vi "VI Algebraic Konfig.vi"() -> ()   [LabVIEW 2020, in "FT-IR.lvlib" / "Algebraic Modul.lvlib"]
uses:
  Algebraic Modul.lvlib
  Visualisierungs Elemente/Button.ctl
  FGV Algebraic Aktionen.ctl
  Messdaten/Aktionen FGV Messdaten.ctl
  FGV FT-IR Gasliste Aktionen.ctl
  FT-IR.lvlib
  Messdaten/Messdaten.lvlib
  Log Konfig/LogKonfig.lvlib
  Allgemein/allgemeine Sub-VIs.lvlib
panel:
  out "OK?":bool[](array[boolean]) caption="Gültig?"
  in  "Abbrechen":T1
  out "Aktuelle Gasliste":string[](array[string])
  in  "Formel":string[](array[string])
  in  "Namen":string[](array[string])
  in  "Speichern":T1
  # "Algebraic Konfiguration"
  # "Gasliste"
  # "Name"
  # "Formel"
  # "Gültig?"
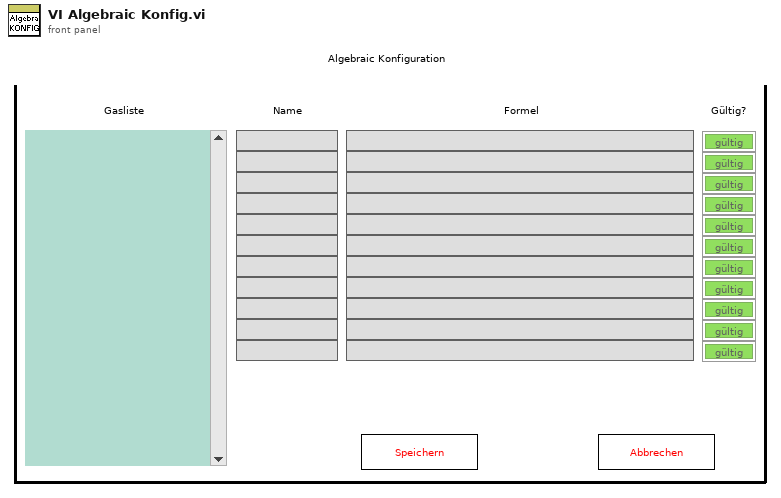
[diagram p1: front panel]
types:
  T1 = typedef "Button.ctl" = bool
  T2 = typedef "FT-IR.lvlib/FGV FT-IR Gasliste Aktionen.ctl" = enum16{"lesen", "Gasliste FT-IR", "Gasliste ausgelesen", "laden", "speichern", "löschen"}
  T3 = typedef "Messdaten.lvlib/Aktionen FGV Messdaten.ctl" = enum16{"lesen", "schreiben", "löschen", "Mittelwerte", "Komponente"}
  T4 = typedef "FT-IR.lvlib/Algebraic Modul.lvlib/FGV Algebraic Aktionen.ctl" = enum16{"lesen", "laden", "speichern", "berechnen", "schreiben"}
  T5 = typedef "String - Ausgabefeld.ctl" = string
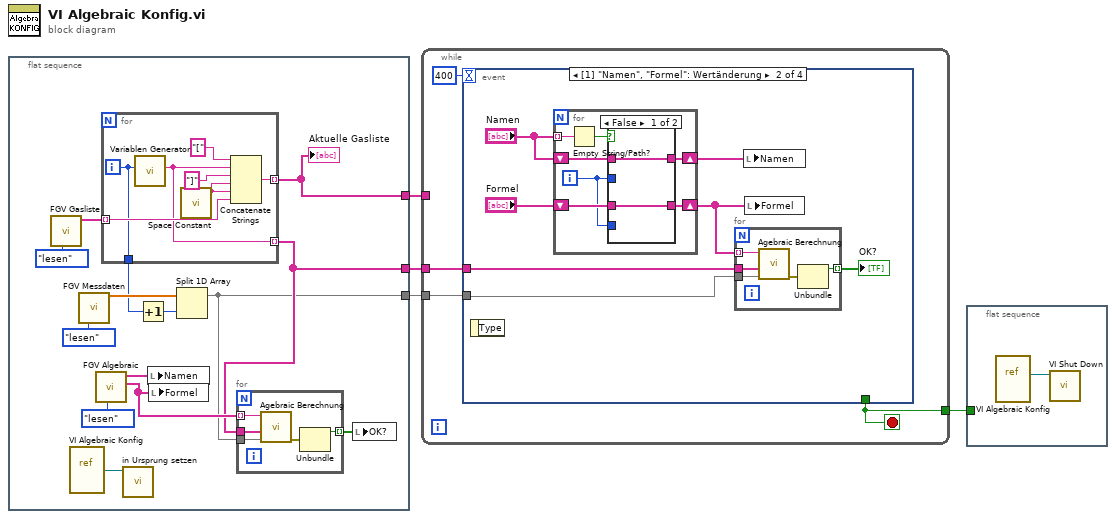
[diagram p0: block diagram]
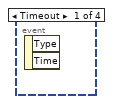
[diagram p2: hidden frame]
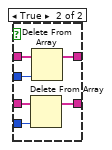
[diagram p3: hidden frame]
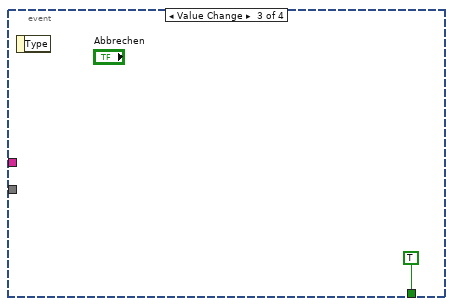
[diagram p4: hidden frame]
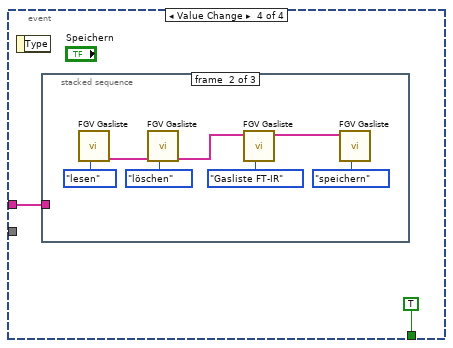
[diagram p5: hidden frame]
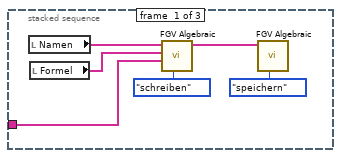
[diagram p6: hidden frame]
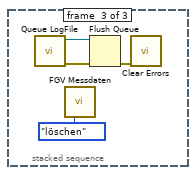
[diagram p7: hidden frame]
diagram:
  n1 = flat-sequence {
    tunnel: [w17] -> w4
    tunnel: [w12] -> w3
    tunnel: [w8] -> w1
    frame #0 {
      n2 = call "FGV Gasliste.vi"("Aktionen"=FGV_FT-IR_Gasliste_Aktionen."lesen") -> ("Aktuelle Gasliste FT-IR"=w18:T5[])  [unwired: 8 in, 2 out]
      n3 = vi-ref "VI Algebraic Konfig.vi"() -> (w5:refnum<vi>)
      n4 = call "FGV Messdaten.vi"("Aktionen"=Aktionen_FGV_Messdaten."lesen") -> ("Aktuelle Messwerte"=w9:sgl[])  [unwired: 6 in, 8 out]
      n5 = call "FGV Algebraic.vi"("Aktionen Algebraic"=FGV_Algebraic_Aktionen."lesen") -> ("Formel"=w13:string[], "Namen"=w15:string[])  [unwired: 6 in, 3 out]
      n6 = for {
        tunnel: w18 -> [w27] mode=indexing
        tunnel: [w28] -> w17 mode=indexing
        tunnel: [w24] -> w12 mode=indexing
        tunnel: [w25] -> w7
        i -> [w25]
        n7 = call "Variablen Generator.vi"("Numerisch"=w25) -> ("Verknüpfter String"=w24:string)  [unwired: 10 in]
        n8 = call <vilib>:"Space Constant.vi"() -> ("String"=w26:string)
        n9 = Concatenate Strings("[" ("String"), w24, "]" ("String"), w26, w26, w27) -> (w28:string)
      }
      "Aktuelle Gasliste" <- w17
      n10 = call "in Ursprung setzen.vi"("VI Referenz"=w5) -> ()  [unwired: 10 in, 1 out]
      n11 = Increment(x=w7) -> (x+1=w6:i32)
      n12 = local write "Namen"(w15) -> ()
      n13 = local write "Formel"(w13) -> ()
      n14 = Split 1D Array(array=w9, index=w6) -> (first subarray=w8:sgl[])  [unwired: 1 out]
      n15 = for {
        tunnel: w13 -> [w23] mode=indexing
        tunnel: w12 -> [w22]
        tunnel: [w20] -> w14 mode=indexing
        tunnel: w8 -> [w19]
        n16 = call "Agebraic Berechnung.vi"("X Values"=w19, "Variables"=w22, "formula"=w23) -> ("error out"=w21:errorcluster)  [unwired: 7 in, 1 out]
        n17 = Unbundle(w21) -> ("status"=w20:bool)  [unwired: 2 out]
      }
      n18 = local write "OK?"(w14) -> ()
    }
  }
  n19 = while {
    tunnel: w4 -> [_]
    tunnel: w3 -> [w33]
    tunnel: [w32] -> w2
    tunnel: w1 -> [w31]
    stop <- w32 stop-if-true
    n20 = event shown="[1] \"Namen\", \"Formel\": Wertänderung" {
      selector: _ -> [_ _ _ _]
      dyn-events: _ -> [_ _ _ _]
      timeout: 400 -> [_ _ _ _]
      tunnel: [_ _ TRUE TRUE] -> w32
      tunnel: w33 -> [_ w38 _ w63]
      tunnel: w31 -> [_ w36 _ _]
      event Timeout {
        n21 = event-data() -> ()  [unwired: 1 in, 2 out]
      }
      event "Namen", "Formel": Value Change {
        n22 = event-data() -> ()  [unwired: 1 in, 1 out]
        n23 = for {
          tunnel: "Namen" -> [w53] mode=indexing
          shift-right: [w51] -> w40
          shift-left: "Namen" -> [w52]
          shift-right: [w49] -> w39
          shift-left: "Formel" -> [w48]
          i -> [w47]
          n24 = Empty String/Path?(string/path=w53) -> (empty?=w50:bool)
          n25 = case shown="False" w50 {
            tunnel: w52 -> [w55 w61]
            tunnel: [w55 w60] -> w51
            tunnel: w47 -> [_ w59]
            tunnel: [w54 w58] -> w49
            tunnel: w48 -> [w54 w57]
            tunnel: w47 -> [_ w56]
            frame False {
            }
            frame True {
              n26 = Delete From Array(array=w57, index=w56) -> (array with subset deleted=w58:string[])  [unwired: 1 in, 1 out]
              n27 = Delete From Array(array=w61, index=w59) -> (array with subset deleted=w60:string[])  [unwired: 1 in, 1 out]
            }
          }
        }
        n28 = for {
          tunnel: w39 -> [w46] mode=indexing
          tunnel: w38 -> [w45]
          tunnel: [w44] -> w37 mode=indexing
          tunnel: w36 -> [w43]
          n29 = call "Agebraic Berechnung.vi"("X Values"=w43, "Variables"=w45, "formula"=w46) -> ("error out"=w42:errorcluster)  [unwired: 7 in, 1 out]
          n30 = Unbundle(w42) -> ("status"=w44:bool)  [unwired: 2 out]
        }
        "OK?" <- w37
        n31 = local write "Namen"(w40) -> ()
        n32 = local write "Formel"(w39) -> ()
      }
      event Value Change {
        n33 = event-data() -> ()  [unwired: 1 in, 1 out]
      }
      event Value Change {
        n34 = event-data() -> ()  [unwired: 1 in, 1 out]
        n35 = stacked-sequence {
          tunnel: w63 -> [w67 _ _]
          frame #0 {
            n36 = local read "Namen"() -> (w69:string[])
            n37 = local read "Formel"() -> (w68:string[])
            n38 = call "FGV Algebraic.vi"("Aktionen Algebraic"=FGV_Algebraic_Aktionen."schreiben", "Variablen"=w67, "Formel"=w68, "Namen"=w69) -> ("Namen"=w65:string[])  [unwired: 3 in, 4 out]
            n39 = call "FGV Algebraic.vi"("Aktionen Algebraic"=FGV_Algebraic_Aktionen."speichern", "Namen"=w65) -> ()  [unwired: 5 in, 5 out]
          }
          frame #1 {
            n40 = call "FGV Gasliste.vi"("Aktionen"=FGV_FT-IR_Gasliste_Aktionen."lesen") -> ("Gasliste ausgelesen"=w71:T5[])  [unwired: 8 in, 2 out]
            n41 = call "FGV Gasliste.vi"("Aktionen"=FGV_FT-IR_Gasliste_Aktionen."löschen", "Gasliste ausgelesen"=w71) -> ("Gasliste ausgelesen"=w73:T5[])  [unwired: 7 in, 2 out]
            n42 = call "FGV Gasliste.vi"("Aktionen"=FGV_FT-IR_Gasliste_Aktionen."Gasliste FT-IR", "Aktuelle Gasliste FT-IR"=w73) -> ("Aktuelle Gasliste FT-IR"=w75:T5[])  [unwired: 7 in, 2 out]
            n43 = call "FGV Gasliste.vi"("Aktionen"=FGV_FT-IR_Gasliste_Aktionen."speichern", "Aktuelle Gasliste FT-IR"=w75) -> ()  [unwired: 7 in, 3 out]
          }
          frame #2 {
            n44 = call "Queue LogFile.vi"() -> ("error out"=w81:errorcluster, "Queue (Ausgang)"=w80:refnum<queue>)  [unwired: 6 in]
            n45 = call "FGV Messdaten.vi"("Aktionen"=Aktionen_FGV_Messdaten."löschen") -> ()  [unwired: 6 in, 9 out]
            n46 = Flush Queue(queue=w80, error in (no error)=w81) -> (error out=w78:errorcluster)  [unwired: 2 out]
            n47 = call <vilib>:"Clear Errors.vi"("error in (no error)"=w78) -> ()  [unwired: 5 in, 2 out]
          }
        }
      }
    }
  }
  n48 = flat-sequence {
    tunnel: w2 -> [_]
    frame #0 {
      n49 = vi-ref "VI Algebraic Konfig.vi"() -> (w82:refnum<vi>)
      n50 = call "VI Shut Down.vi"("VI Referenz"=w82) -> ()  [unwired: 11 in]
    }
  }
